vi "init_currentDAQ_v01.vi"(5 "protocol waveform":dbl[](graph), 6 "Duration (s)":dbl, 7 "Sample Freq (Hz)":dbl min=0.0 max=40000.0, 8 "AO error in":errorcluster, 9 "AO physical channels":tag="cDAQ1Mod3/ao14", 10 "AI error in":errorcluster, 11 "AI Physical Channel":tag="cDAQ1Mod1/ai0") -> (0 "AO error out":errorcluster, 1 "AO task out":refnum<k21>, 2 "AI error out":errorcluster, 3 "AI task out":refnum<k21>, 4 "protocol response":dbl[](graph) caption="jumptestMonitor")   [LabVIEW 2019]
uses:
  <vilib>/DAQmx/write.llb/DAQmx Write (Analog Wfm 1Chan NSamp).vi
  <vilib>/DAQmx/create/channels.llb/DAQmx Create Channel (AO-Voltage-Basic).vi
  <vilib>/DAQmx/configure/timing.llb/DAQmx Timing (Sample Clock).vi
  <vilib>/DAQmx/create/channels.llb/DAQmx Create Channel (AI-Voltage-Basic).vi
  <vilib>/DAQmx/configure/trigger.llb/DAQmx Start Trigger (Digital Edge).vi
  <vilib>/DAQmx/miscellaneous.llb/DAQmx Fill In Error Info.vi
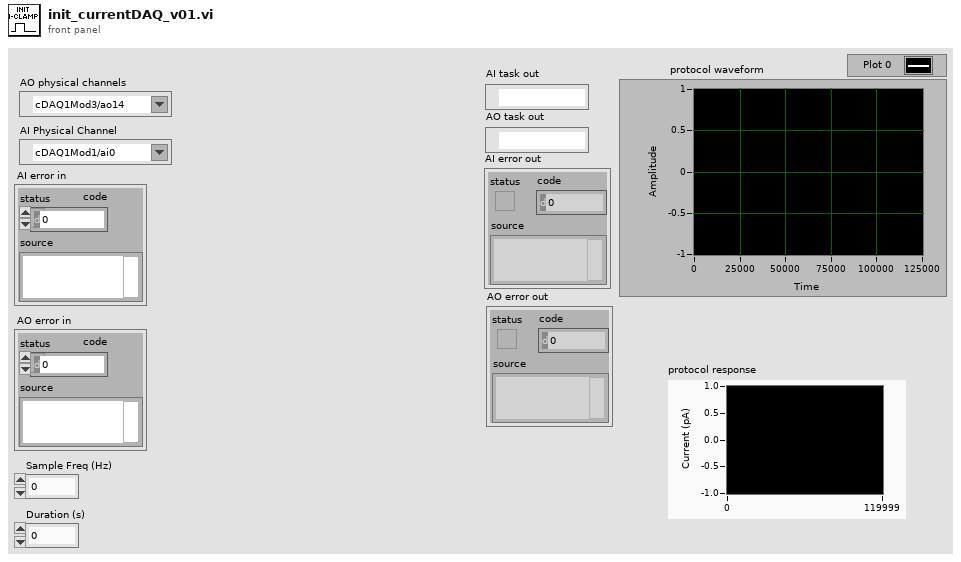
[diagram p1: front panel]
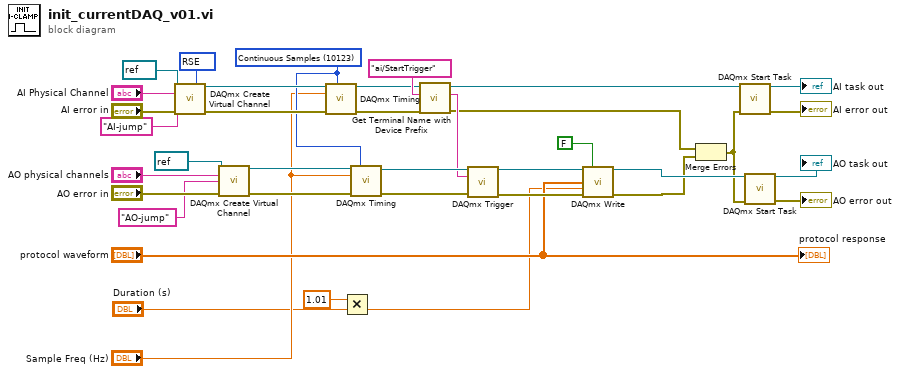
[diagram p0: block diagram]
diagram:
  w34 = 10083 items=["default"=-1, "RSE"=10083, "NRSE"=10078, "Differential"=10106, "Pseudodifferential"=12529] ("input terminal configuration")
  w25 = 10123 items=["Finite Samples"=10178, "Continuous Samples"=10123] ("sample mode")
  n1 = call-poly <vilib>:"DAQmx Create Virtual Channel.vi"("task in"=refnum<k21> refnum, "input terminal configuration"=w34, "physical channels"="AI Physical Channel", "name to assign"="AI-jump", "error in"="AI error in") -> ("task out"=w36:refnum<k21>, "error out"=w37:errorcluster)  [unwired: 9 in]
  n2 = call-poly <vilib>:"DAQmx Create Virtual Channel.vi"("task in"=refnum<k21> refnum, "physical channels"="AO physical channels", "name to assign"="AO-jump", "error in"="AO error in") -> ("task out"=w27:refnum<k21>, "error out"=w26:errorcluster)  [unwired: 10 in]
  n3 = call-poly <vilib>:"DAQmx Timing.vi"("task/channels in"=w36, "sample mode"=w25, "rate"="Sample Freq (Hz)", "error in"=w37) -> ("task out"=w31:refnum<k21>, "error out"=w30:errorcluster)  [unwired: 10 in]
  n4 = Multiply(x=1.01, y="Duration (s)") -> (x*y=w2:dbl)
  n5 = call-poly <vilib>:"DAQmx Timing.vi"("task/channels in"=w27, "sample mode"=w25, "rate"="Sample Freq (Hz)", "error in"=w26) -> ("task out"=w23:refnum<k21>, "error out"=w24:errorcluster)  [unwired: 10 in]
  n6 = call "Get Terminal Name with Device Prefix.vi"("error in (no error)"=w30, "Local Terminal Name"="ai/StartTrigger" ("terminal"), "task/channels in"=w31) -> ("error out"=w19:errorcluster, "Terminal Name with Device Prefix"=w22:tag, "task out"=w16:refnum<k21>)  [unwired: 6 in]
  n7 = call-poly <vilib>:"DAQmx Trigger.vi"("task/channels in"=w23, "source"=w22, "error in"=w24) -> ("task out"=w21:refnum<k21>, "error out"=w20:errorcluster)  [unwired: 11 in]
  n8 = call-poly <vilib>:"DAQmx Write.vi"("task/channels in"=w21, "auto start"=FALSE, "data"="protocol waveform", "timeout"=w2, "error in"=w20) -> ("task out"=w17:refnum<k21>, "error out"=w5:errorcluster)  [unwired: 8 in, 1 out]
  n9 = Merge Errors(w19, w5) -> (w4:errorcluster)
  n10 = call <vilib>:"DAQmx Start Task.vi"("task/channels in"=w16, "error in"=w4) -> ("task out"=→"AI task out":refnum<k21>, "error out"=→"AI error out":errorcluster)  [unwired: 12 in]
  n11 = call <vilib>:"DAQmx Start Task.vi"("task/channels in"=w17, "error in"=w4) -> ("task out"=→"AO task out":refnum<k21>, "error out"=→"AO error out":errorcluster)  [unwired: 12 in]
  "protocol response" <- "protocol waveform"
